vi "Set Gain.vi"(8 "error in (no error)":errorcluster, 10 "Gain":u8 step=1, 11 "Hamamatsu_Camera in":refnum<class "Hamamatsu_Camera.lvclass">) -> (0 "error out":errorcluster, 3 "Hamamatsu_Camera out":refnum<class "Hamamatsu_Camera.lvclass">)   [LabVIEW 2023, in "Hamamatsu_Camera.lvlib" / "Hamamatsu_Camera.lvclass"]
uses:
  Hamamatsu_Camera.lvclass
  Hamamatsu_Camera.lvclass/Hamamatsu_Camera.ctl
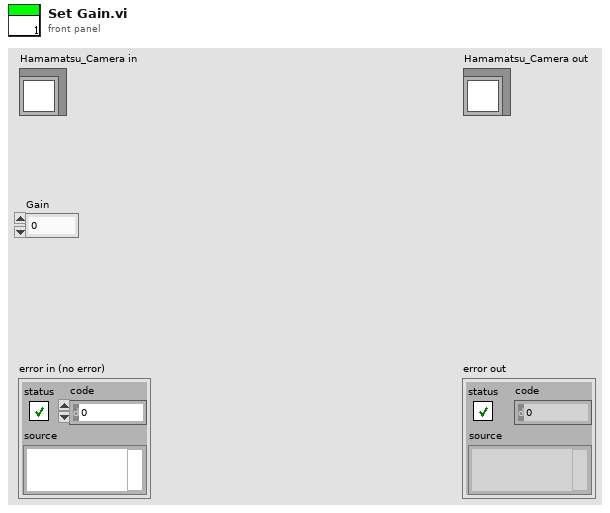
[diagram p1: front panel]
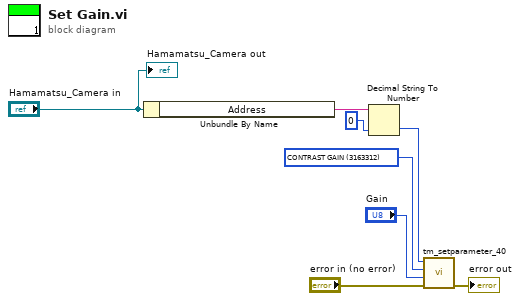
[diagram p0: block diagram]
diagram:
  w8 = u32 3163312 items=["SENSOR MODE"=4212128, "SENSOR MODE LINE BUNDLE HEIGHT"=4212192, "READOUT DIRECTION"=4211904, "BIT PER CHANNEL"=4342976, "EXPOSURE TIME"=2049184, "CONTRAST GAIN"=3163312, "BINNING"=4215968, "TIMING READOUT TIME"=4223904, "INTERNAL FRAME RATE"=4225952, "INTERNAL FRAME INTERVAL"=4225968, "INTERNAL LINE SPEED"=4226000, "IMAGE WIDTH"=4343200, "IMAGE HEIGHT"=4343216, "IMAGE ROWBYTES"=4343232, "IMAGE FRAMEBYTES"=4343248, "IMAGE PIXEL TYPE"=4343296] ("Parameter")
  n1 = Unbundle By Name("Hamamatsu_Camera in") -> ("Address"=w6:string)
  n2 = Decimal String To Number(string=w6, default (0L)=u32 0 ("default (0 I32)")) -> (number=w3:u32)  [unwired: 1 in, 1 out]
  n3 = call "tm_setparameter_40.vi"("error in (no error)"="error in (no error)", "Value in"="Gain", "Parameter"=w8, "Handle in"=w3) -> ("error out"=→"error out":errorcluster)  [unwired: 6 in, 1 out]
  "Hamamatsu_Camera out" <- "Hamamatsu_Camera in"
